vi "IncrementNumber.vi"(11 "ExampleClass in":refnum<class "ExampleClass.lvclass">) -> (3 "ExampleClass out":refnum<class "ExampleClass.lvclass">)   [LabVIEW 2012, in "ExampleClass.lvclass"]
uses:
  ExampleClass.lvclass
  ExampleClass.lvclass/ExampleClass.ctl
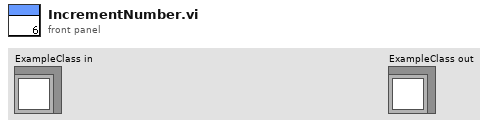
[diagram p1: front panel]
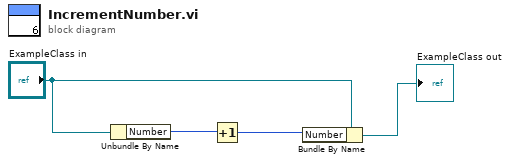
[diagram p0: block diagram]
diagram:
  n1 = Unbundle By Name("ExampleClass in") -> ("Number"=w3:i32)
  n2 = Increment(x=w3) -> (x+1=w2:i32)
  n3 = Bundle By Name(cluster="ExampleClass in", "Number"=w2) -> (→"ExampleClass out":refnum<class "ExampleClass.lvclass">)
